vi "Get Server Stop UE.vi"(11 "OOP Server in":refnum<class "Ex1_server.lvclass">) -> (2 "Server Stop":refnum<user-event>, 3 "OOP Server out":refnum<class "Ex1_server.lvclass">)   [LabVIEW 2019, in "Ex1_server.lvlib" / "Ex1_server.lvclass"]
uses:
  Ex1_server.lvclass
  Ex1_server.lvclass/Ex1_server.ctl
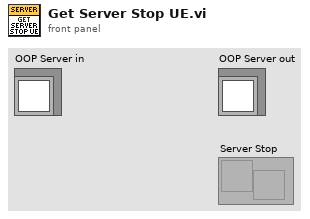
[diagram p1: front panel]
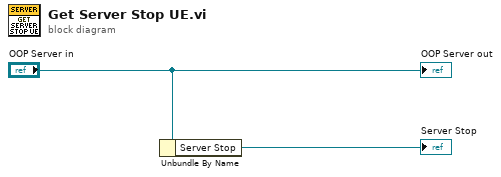
[diagram p0: block diagram]
diagram:
  n1 = Unbundle By Name("OOP Server in") -> ("Server Stop"=→"Server Stop":refnum<user-event>)
  "OOP Server out" <- "OOP Server in"
